vi "first FPGA PC.vi"() -> ()   [LabVIEW 2018]
uses:
  <vilib>/Math Plots/2D Math Plots/2D Error Bar/2D Error Bar XCtrl/2D Error Bar.xctl
panel:
  in  "length":i32
  in  "2D array":dbl[][](array[numeric])
  out "2D Error Bar":refnum<class "2D Plot Datatype.lvclass">[](xcontrol)
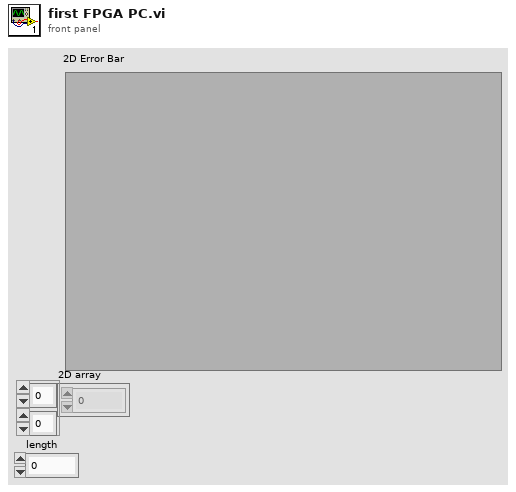
[diagram p1: front panel]
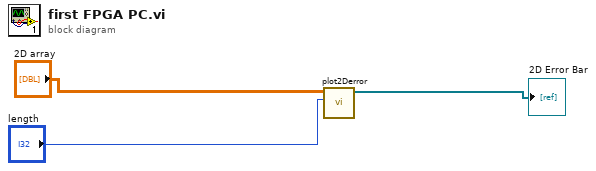
[diagram p0: block diagram]
diagram:
  n1 = call "plot2Derror.vi"("length"="length", "2D array"="2D array") -> ("2D Error Bar"=→"2D Error Bar":refnum<class "2D Plot Datatype.lvclass">[])  [unwired: 9 in]
